vi "Read SSF.vi"(8 "error in (no error)":errorcluster, 11 "SSF Path":path) -> (0 "error out":errorcluster, 1 "Test Case Order":T1, 2 "Product Data":T3, 3 "Station Data":T2)   [LabVIEW 2024]
doc: "Reads back station, product and test order data from .ssf (config) file."
uses:
  Product Data.ctl
  Station Data.ctl
  Test Case Order.ctl
  <vilib>/Utility/config.llb/NI_LVConfig.lvlib
  <userlib>/_OpenG.lib/variantconfig/variantconfig.llb/openg_variant_configuration_file.lvlib
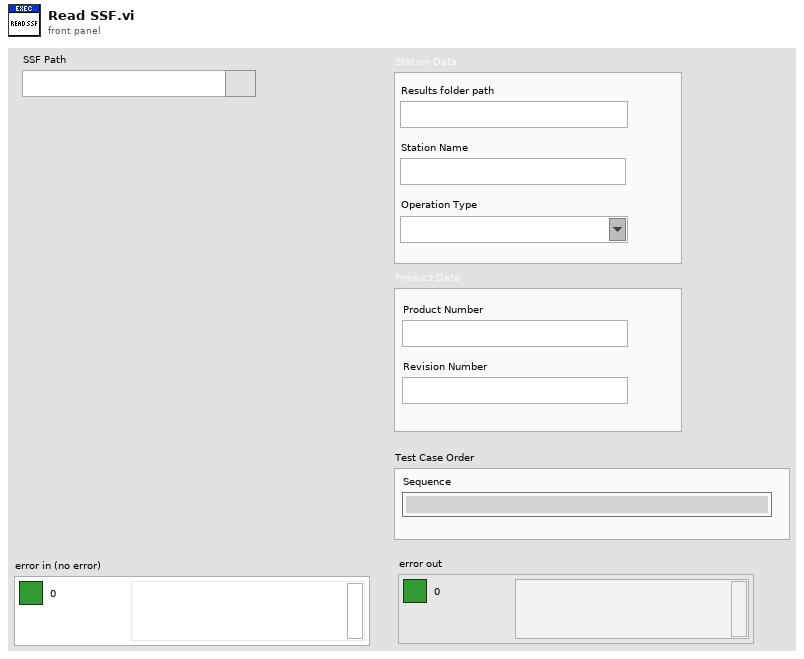
[diagram p1: front panel]
types:
  T1 = typedef "Test Case Order.ctl" = cluster{"Sequence":string}
  T2 = typedef "Station Data.ctl" = cluster{"Results folder path":path, "Station Name":string, "Operation Type":string}
  T3 = typedef "Product Data.ctl" = cluster{"Product Number":string, "Revision Number":string}
  T4 = typedef "NI_LVConfig.lvlib/Config Data RefNum.ctl" = refnum<k1>
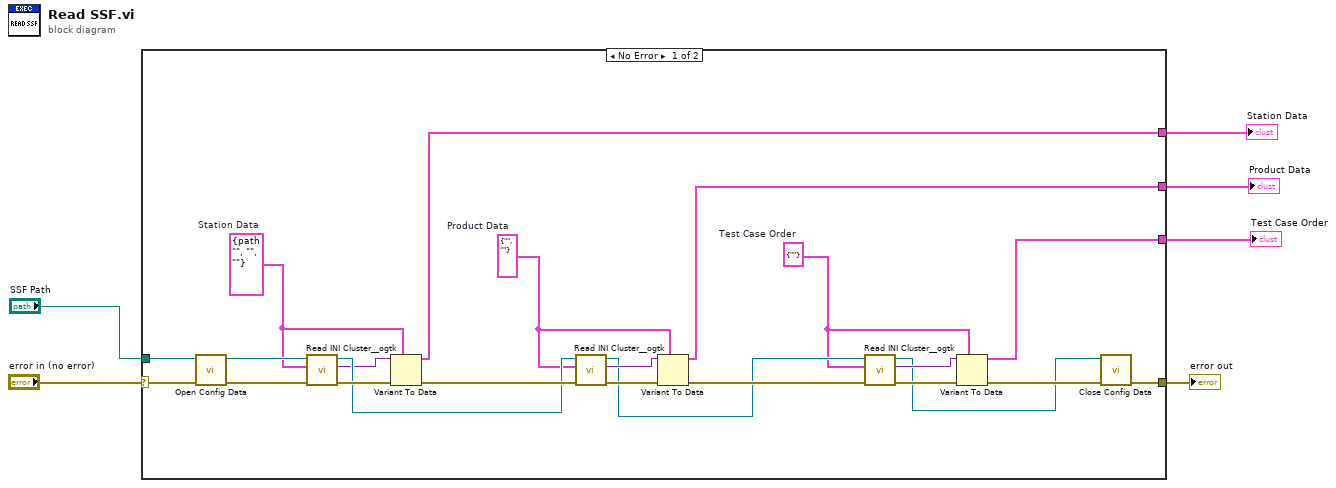
[diagram p0: block diagram]
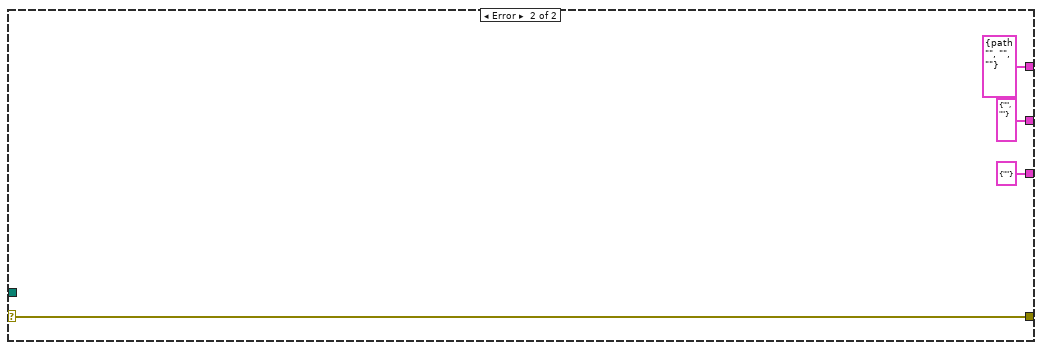
[diagram p2: hidden frame]
diagram:
  n1 = case shown="No Error" "error in (no error)" {
    selector: "error in (no error)" -> [w29 w33]
    tunnel: [w7 w33] -> w6
    tunnel: "SSF Path" -> [w28 _]
    tunnel: [w10 T2 {"Results folder path"=path "", "Station Name"="", "Operation Type"=""} ("Station Data")] -> w3
    tunnel: [w9 T1 {"Sequence"=""} ("Test Case Order")] -> w2
    tunnel: [w8 T3 {"Product Number"="", "Revision Number"=""} ("Product Data")] -> w1
    frame No Error {
      w11 = T1 {"Sequence"=""}  # Test Case Order
      w18 = T2 {"Results folder path"=path "", "Station Name"="", "Operation Type"=""}  # Station Data
      w21 = T3 {"Product Number"="", "Revision Number"=""}  # Product Data
      n2 = call <vilib>:"Open Config Data.vi"("error in (no error)"=w29, "configuration file path"=w28) -> ("error out"=w20:errorcluster, "refnum"=w19:T4)  [unwired: 7 in, 1 out]
      n3 = call <userlib>:"Read INI Cluster__ogtk.vi"("error in (no error)"=w20, "INI Fomatted Cluster Type"=w18, "refnum"=w19) -> ("error out"=w27:errorcluster, "INI Fomatted Cluster"=w24:variant, "dup refnum"=w25:T4)  [unwired: 4 in, 2 out]
      n4 = Variant To Data(error in=w27, type=w18, Variant=w24) -> (data=w10:T2, error out=w26:errorcluster)
      n5 = call <userlib>:"Read INI Cluster__ogtk.vi"("error in (no error)"=w26, "INI Fomatted Cluster Type"=w21, "refnum"=w25) -> ("error out"=w23:errorcluster, "INI Fomatted Cluster"=w22:variant, "dup refnum"=w12:T4)  [unwired: 4 in, 2 out]
      n6 = Variant To Data(error in=w23, type=w21, Variant=w22) -> (data=w8:T3, error out=w16:errorcluster)
      n7 = call <userlib>:"Read INI Cluster__ogtk.vi"("error in (no error)"=w16, "INI Fomatted Cluster Type"=w11, "refnum"=w12) -> ("error out"=w15:errorcluster, "INI Fomatted Cluster"=w17:variant, "dup refnum"=w13:T4)  [unwired: 4 in, 2 out]
      n8 = Variant To Data(error in=w15, type=w11, Variant=w17) -> (data=w9:T1, error out=w14:errorcluster)
      n9 = call <vilib>:"Close Config Data.vi"("error in (no error)"=w14, "refnum"=w13) -> ("error out"=w7:errorcluster)  [unwired: 8 in, 1 out]
    }
    frame Error {
    }
  }
  "error out" <- w6
  "Product Data" <- w1
  "Test Case Order" <- w2
  "Station Data" <- w3
